vi "Initialize UI Loop.vi"(8 "error in":errorcluster, 11 "UI Data in":T1 {"SR Display List"."Creation Date" format="%<%x>T"; "SR Display List"."Last Updated" format="%<%x>T"}) -> (0 "error out":errorcluster, 3 "UI Data out 2":T1 {"SR Display List"."Creation Date" format="%<%x>T"; "SR Display List"."Last Updated" format="%<%x>T"})   [LabVIEW 2018]
uses:
  Type Defs/UI Loop Data.ctl
  Type Defs/SR Cluster.ctl
  Type Defs/SR Status.ctl
  Type Defs/Filter Cluster.ctl
  Type Defs/Sorting Methods.ctl
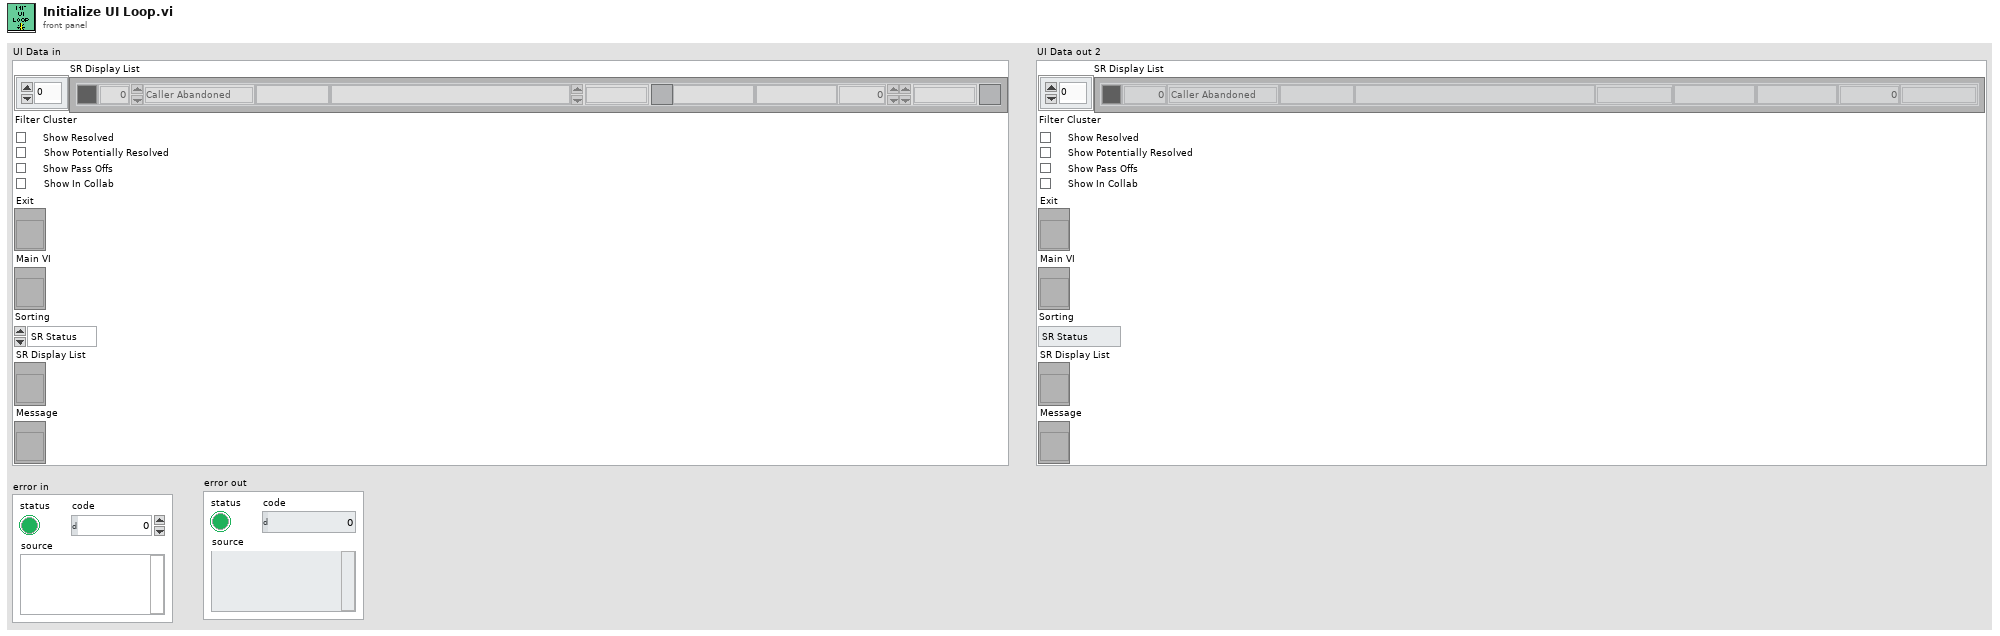
[diagram p1: front panel]
types:
  T1 = typedef "UI Loop Data.ctl" = cluster{"SR Display List":T2[], "Filter Cluster":T4, "Exit":refnum<vi>, "Main VI":refnum<vi>, "Sorting":T5, "SR Display List":refnum<vi>, "Message":refnum<vi>}
  T2 = typedef "SR Cluster.ctl" = cluster{"Color":u32, "SR Number":i32, "SR Status":T3, "Name":string, "Summary":string, "Last Updated":timestamp, "SR Type":string, "Service Level":string, "Days Open":dbl, "Creation Date":timestamp}
  T3 = typedef "SR Status.ctl" = enum16{"Caller Abandoned", "Created in Error", "Expired", "Forum Resolved AE", "Forum Resolved Customer", "IN WORK", "IN WORK Collab with AES", "IN WORK Collab with PSE", "IN WORK Collab with SE", "IN WORK Customer Added Note", "IN WORK Escalation", "IN WORK Wait on Customer", "Open", "Potentially Resolved", "Presumed Resolved", "RMA Approved for Return", "Resolved", "Passed Off"}
  T4 = typedef "Filter Cluster.ctl" = cluster{"Show Resolved":bool, "Show Potentially Resolved":bool, "Show Passoffs":bool, "Show In Collab":bool}
  T5 = typedef "Sorting Methods.ctl" = enum16{"SR Status", "Most Recent", "SR Type", "SR Number"}
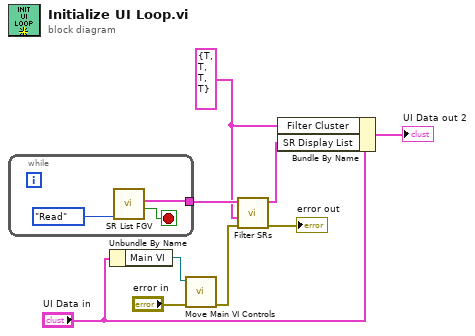
[diagram p0: block diagram]
diagram:
  w6 = T4 {"Show Resolved"=TRUE, "Show Potentially Resolved"=TRUE, "Show Passoffs"=TRUE, "Show In Collab"=TRUE} ("Filter Cluster")
  n1 = while {
    tunnel: [w11] -> w9
    stop <- w12 stop-if-true
    n2 = call "SR List FGV.vi"("Operation"=enum16{"Initialize", "Write", "Read", "Clear"}."Read") -> ("Updated?"=w12:bool, "list out"=w11:T2[])  [unwired: 9 in]
  }
  n3 = Unbundle By Name("UI Data in") -> ("Main VI"=w5:refnum<vi>)
  n4 = call "Move Main VI Controls.vi"("error in"="error in", "VIRef in"=w5) -> ("error out"=w8:errorcluster)  [unwired: 9 in]
  n5 = call "Filter SRs.vi"("error in"=w8, "Filter Cluster"=w6, "list in"=w9) -> ("error out"=→"error out":errorcluster, "list out"=w7:T2[])  [unwired: 7 in]
  n6 = Bundle By Name(cluster="UI Data in", "Filter Cluster"=w6, "SR Display List"=w7) -> (→"UI Data out 2":T1)
